vi "(SubVI) Read All Data _YCC.vi"(7 "Folder Path":path) -> (1 "all moved time points":dbl[](array[numeric]), 2 "all QPD data":dbl[](array[numeric]), 3 "Last File Path":path)   [LabVIEW 2014]
uses:
  <vilib>/Utility/file.llb/Read From Spreadsheet File (DBL).vi
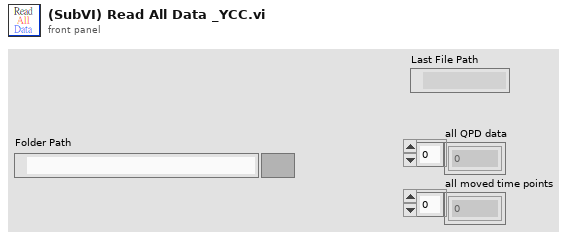
[diagram p1: front panel]
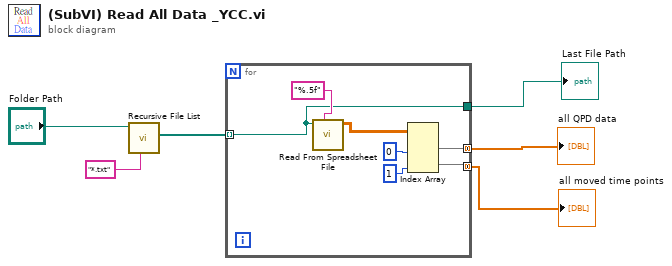
[diagram p0: block diagram]
diagram:
  n1 = call <vilib>:"Recursive File List.vi"("pattern"="*.txt", "Folder Path"="Folder Path") -> ("All Files in Dir"=w4:path[])  [unwired: 5 in, 4 out]
  n2 = for {
    tunnel: w4 -> [w7] mode=indexing
    tunnel: [w9] -> w3 mode=concatenating
    tunnel: [w8] -> w2 mode=concatenating
    tunnel: [w7] -> w1
    n3 = call-poly <vilib>:"Read From Spreadsheet File.vi"("format (%.3f)"="%.5f", "file path (dialog if empty)"=w7) -> ("all rows"=w10:dbl[][])  [unwired: 5 in, 4 out]
    n4 = Index Array(array=w10, index (col) #1=0 ("disabled index (col)"), index (col) #2=1 ("index (col)")) -> (element #1=w9:dbl[], element #2=w8:dbl[])  [unwired: 2 in]
  }
  "all QPD data" <- w3
  "all moved time points" <- w2
  "Last File Path" <- w1
